vi "dataAcquisitionLoop.vi"(1 "total time":dbl format="%#_13g") -> (0 "Data Cluster":T1)   [LabVIEW 2013]
uses:
  <vilib>/Platform/TimedLoop/XDataNode/timing_clust.ctl
  <vilib>/Platform/TimedLoop/XDataNode/nitl_modes.ctl
  <vilib>/Platform/TimedLoop/XDataNode/wakeup.ctl
  <vilib>/DAQmx/read.llb/DAQmx Read (Analog 1D DBL NChan 1Samp).vi
  Global Variables.vi
  <vilib>/DAQmx/create/channels.llb/DAQmx Create Channel (AI-Voltage-Basic).vi
  <vilib>/DAQmx/configure/timing.llb/DAQmx Timing (Sample Clock).vi
  <vilib>/DAQmx/miscellaneous.llb/DAQmx Fill In Error Info.vi
  <vilib>/imath/engines/lvmath2/RunTimeEngine/NodeEndStatement/NIMS_NodeEndStatement_Output.vi
  <instcachedir>/0/NIMS_NodeEndStatement_Output_53EC0D466D134D7ABD903AC30B43404B.lvgen/NIMS_NodeEndStatement_Output_53EC0D466D134D7ABD903AC30B43404B_001.vi
  <vilib>/imath/engines/lvmath2/RunTimeEngine/ErrorHandling/NIMS_Finalize Error.vi
  <vilib>/Platform/TimedLoop/XDataNode/XDataNode.xnode
  <vilib>/Platform/TimedLoop/XDataNode/XDNodeRunTimeDep.lvlib
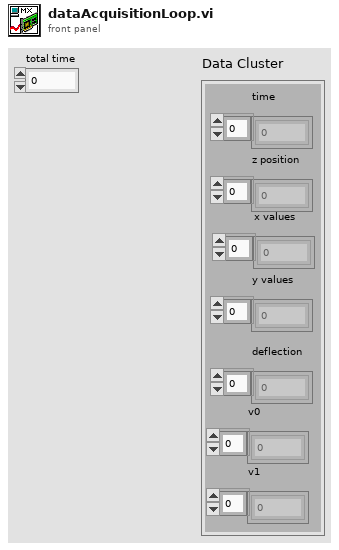
[diagram p1: front panel]
types:
  T1 = cluster{"time":dbl[], "z position":dbl[], "x values":dbl[], "y values":dbl[], "deflection":dbl[], "v0":dbl[], "v1":dbl[]}
  T2 = typedef "XDNodeRunTimeDep.lvlib/timing_clust.ctl" = cluster{"Expected End [f-1]":u64, "Actual End [f-1]":u64, "Finished Late? [f-1]":bool, "Expected End [i-1]":u64, "Actual End [i-1]":u64, "Finished Late? [i-1]":bool, "Expected Start [i]":u64, "Actual Start [i]":u64, "Expected Start [f]":u64, "Actual Start [f]":u64, "Source Name":string, "Structure Name":string, "Period":i64, "Deadline":i64, "Offset":i64, "Start":i64, "Priority":i32, "Timeout":i32, "Mode":T3, "Wakeup Reason":T4, "Error":errorcluster, "Source Type":string, "Secondary Source Type":string, "Global End Time":u64, "Global Start Time":u64, "Frame Duration":u64, "Iteration Duration":u64, "Assigned CPU":i32, "I/O Scan Engine Mode":u32}
  T3 = typedef "XDNodeRunTimeDep.lvlib/nitl_modes.ctl" = enum32{"No Change", "Process missed periods, maintain original phase", "Discard missed periods, maintain original phase", "Process missed periods, ignore original phase", "Discard missed periods, ignore original phase"}
  T4 = typedef "XDNodeRunTimeDep.lvlib/wakeup.ctl" = enum32{"Normal", "Aborted", "Asynchronous wakeup", "Timing source error", "Timed loop error", "Timeout"}
  T5 = cluster{dbl[], "flattned array":dbl[], dbl[], dbl[], "flattned array":dbl[], dbl[], dbl[]}
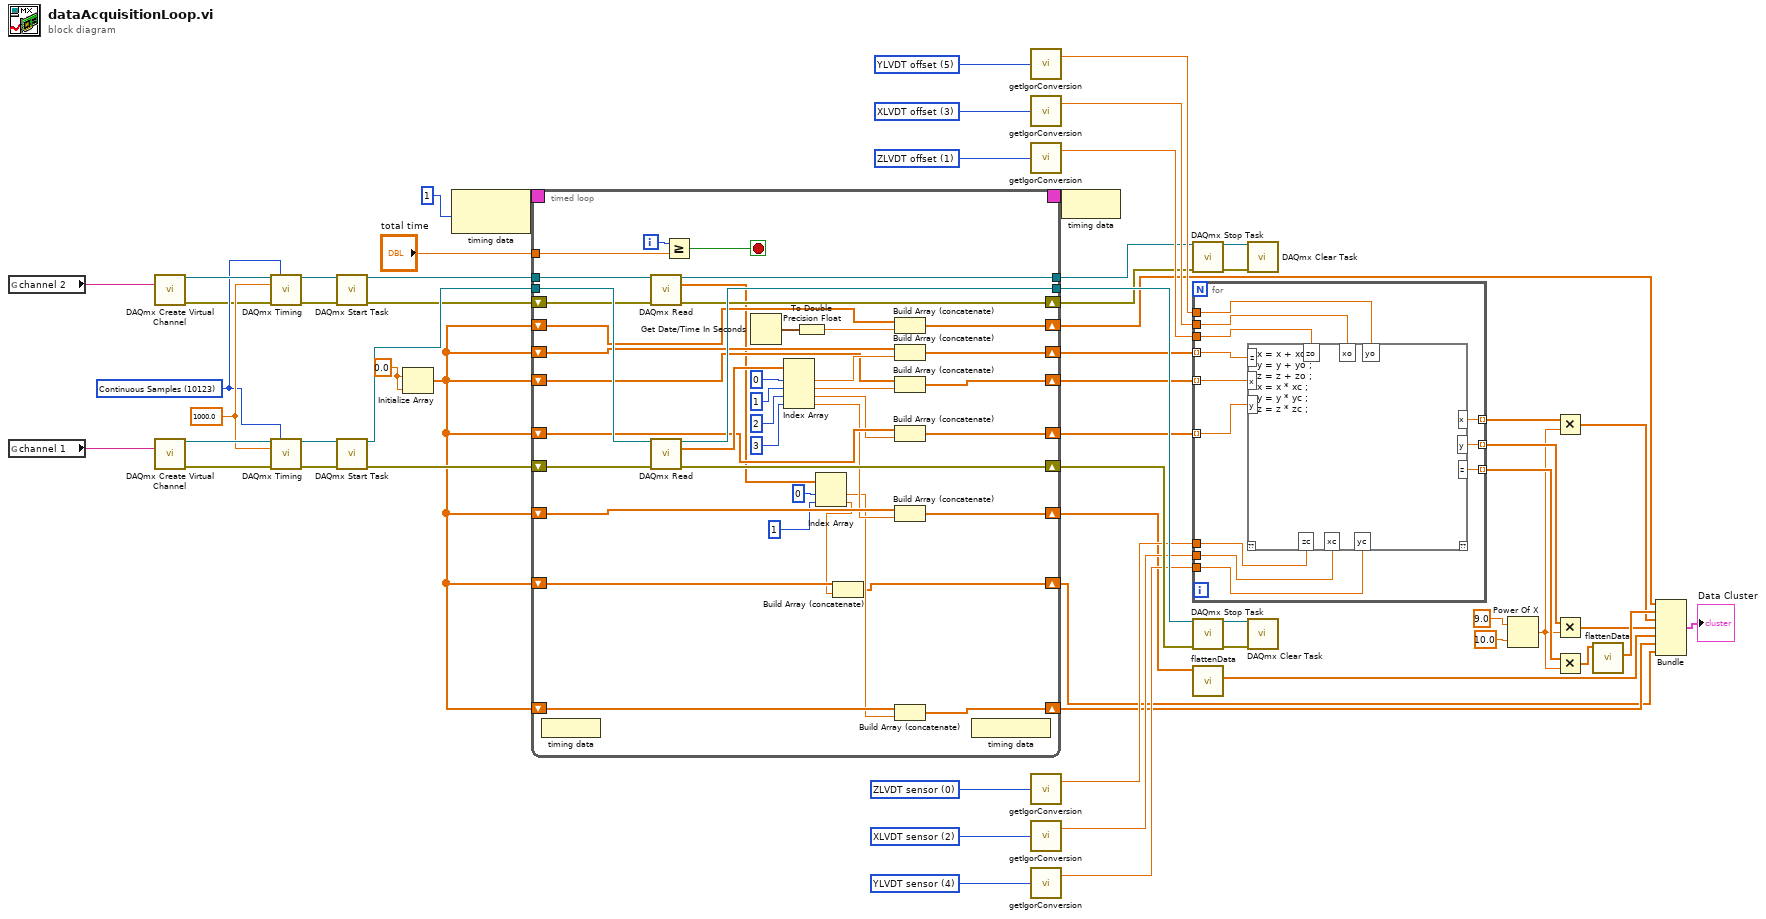
[diagram p0: block diagram]
diagram:
  w27 = 0.0
  w22 = 1000.0
  w34 = 1 items=["ZLVDT sensor", "ZLVDT offset", "XLVDT sensor", "XLVDT offset", "YLVDT sensor", "YLVDT offset", "DEFL"] ("index")
  w33 = 5 items=["ZLVDT sensor", "ZLVDT offset", "XLVDT sensor", "XLVDT offset", "YLVDT sensor", "YLVDT offset", "DEFL"] ("index")
  w32 = 3 items=["ZLVDT sensor", "ZLVDT offset", "XLVDT sensor", "XLVDT offset", "YLVDT sensor", "YLVDT offset", "DEFL"] ("index")
  w39 = 4 items=["ZLVDT sensor", "ZLVDT offset", "XLVDT sensor", "XLVDT offset", "YLVDT sensor", "YLVDT offset", "DEFL"] ("index")
  w38 = 2 items=["ZLVDT sensor", "ZLVDT offset", "XLVDT sensor", "XLVDT offset", "YLVDT sensor", "YLVDT offset", "DEFL"] ("index")
  w37 = 0 items=["ZLVDT sensor", "ZLVDT offset", "XLVDT sensor", "XLVDT offset", "YLVDT sensor", "YLVDT offset", "DEFL"] ("index")
  w19 = 10123 items=["Finite Samples"=10178, "Continuous Samples"=10123, "Hardware Timed Single Point"=12522] ("sample mode")
  n1 = global read "Global Variables.vi" "channel 2"() -> (w21:tag)
  n2 = global read "Global Variables.vi" "channel 1"() -> (w57:tag)
  n3 = call-poly <vilib>:"DAQmx Create Virtual Channel.vi"("physical channels"=w21) -> ("task out"=w20:refnum<k21>, "error out"=w18:errorcluster)  [unwired: 13 in]
  n4 = call-poly <vilib>:"DAQmx Create Virtual Channel.vi"("physical channels"=w57) -> ("task out"=w56:refnum<k21>, "error out"=w51:errorcluster)  [unwired: 13 in]
  n5 = call-poly <vilib>:"DAQmx Timing.vi"("task/channels in"=w20, "sample mode"=w19, "rate"=w22, "error in"=w18) -> ("task out"=w17:refnum<k21>, "error out"=w16:errorcluster)  [unwired: 10 in]
  n6 = call-poly <vilib>:"DAQmx Timing.vi"("task/channels in"=w56, "sample mode"=w19, "rate"=w22, "error in"=w51) -> ("task out"=w55:refnum<k21>, "error out"=w50:errorcluster)  [unwired: 10 in]
  n7 = call <vilib>:"DAQmx Start Task.vi"("task/channels in"=w17, "error in"=w16) -> ("task out"=w15:refnum<k21>, "error out"=w11:errorcluster)  [unwired: 12 in]
  n8 = call <vilib>:"DAQmx Start Task.vi"("task/channels in"=w55, "error in"=w50) -> ("task out"=w54:refnum<k21>, "error out"=w49:errorcluster)  [unwired: 12 in]
  n9 = Initialize Array(w27, w27) -> (w3:dbl[])
  n10 = node-c288(i64 1 ("Period")) -> (w61:T2)
  n11 = timed-loop {
    timing: w61 -> [_]
    timing-out: [_] -> w60
    tunnel: w54 -> [w102]
    tunnel: "total time" -> [w97]
    tunnel: [w101] -> w53
    shift-right: [w99] -> w48
    shift-left: w49 -> [w100]
    shift-right: [w89] -> w26
    shift-left: w3 -> [w90]
    shift-right: [w81] -> w23
    shift-left: w3 -> [w87]
    shift-right: [w79] -> w25
    shift-left: w3 -> [w85]
    shift-right: [w80] -> w24
    shift-left: w3 -> [w86]
    shift-right: [w77] -> w9
    shift-left: w3 -> [w78]
    tunnel: w15 -> [w74]
    tunnel: [w73] -> w13
    shift-right: [w71] -> w10
    shift-left: w11 -> [w72]
    shift-right: [w67] -> w4
    shift-left: w3 -> [w68]
    shift-right: [w62] -> w2
    shift-left: w3 -> [w64]
    i -> [w96]
    stop <- w98 stop-if-true
    n12 = node-c288() -> ()  [unwired: 1 in]
    n13 = call-poly <vilib>:"DAQmx Read.vi"("task/channels in"=w74, "error in"=w72) -> ("task out"=w73:refnum<k21>, "data"=w70:dbl[], "error out"=w71:errorcluster)  [unwired: 11 in]
    n14 = call-poly <vilib>:"DAQmx Read.vi"("task/channels in"=w102, "error in"=w100) -> ("task out"=w101:refnum<k21>, "data"=w95:dbl[], "error out"=w99:errorcluster)  [unwired: 11 in]
    n15 = Greater Or Equal?(x=w96, y=w97) -> (x >= y?=w98:bool)
    n16 = Get Date/Time In Seconds() -> (seconds since 1Jan1904=w76:timestamp)
    n17 = Index Array(array=w95, index #1=0, index #2=1, index #3=2, index #4=3) -> (element #1=w88:dbl, element #2=w84:dbl, element #3=w83:dbl, element #4=w82:dbl)
    n18 = To Double Precision Float(number=w76) -> (double precision float=w75:dbl)
    n19 = Index Array(array=w70, index #1=0, index #2=1) -> (element #1=w66:dbl, element #2=w63:dbl)
    n20 = Build Array (concatenate)(w64, w63) -> (w62:dbl[])
    n21 = Build Array (concatenate)(w78, w75) -> (w77:dbl[])
    n22 = Build Array (concatenate)(w90, w88) -> (w89:dbl[])
    n23 = Build Array (concatenate)(w85, w84) -> (w79:dbl[])
    n24 = Build Array (concatenate)(w86, w83) -> (w80:dbl[])
    n25 = Build Array (concatenate)(w87, w82) -> (w81:dbl[])
    n26 = Build Array (concatenate)(w68, w66) -> (w67:dbl[])
    n27 = node-c288() -> ()  [unwired: 1 out]
  }
  n28 = call "getIgorConversion.vi"("index"=w33) -> ("Result"=w31:dbl)  [unwired: 1 out]
  n29 = call "getIgorConversion.vi"("index"=w32) -> ("Result"=w30:dbl)  [unwired: 1 out]
  n30 = call "getIgorConversion.vi"("index"=w34) -> ("Result"=w29:dbl)  [unwired: 1 out]
  n31 = call "getIgorConversion.vi"("index"=w37) -> ("Result"=w28:dbl)  [unwired: 1 out]
  n32 = call "getIgorConversion.vi"("index"=w38) -> ("Result"=w36:dbl)  [unwired: 1 out]
  n33 = call "getIgorConversion.vi"("index"=w39) -> ("Result"=w35:dbl)  [unwired: 1 out]
  n34 = node-c288(w60) -> ()
  n35 = call <vilib>:"DAQmx Stop Task.vi"("task/channels in"=w13, "error in"=w10) -> ("task out"=w12:refnum<k21>, "error out"=w14:errorcluster)  [unwired: 12 in]
  n36 = for {
    tunnel: w26 -> [w105] mode=indexing
    tunnel: w25 -> [w106] mode=indexing
    tunnel: w24 -> [w107] mode=indexing
    tunnel: [w116] -> w42 mode=indexing
    tunnel: [w115] -> w43 mode=indexing
    tunnel: [w114] -> w44 mode=indexing
    tunnel: w28 -> [w113]
    tunnel: w36 -> [w112]
    tunnel: w35 -> [w111]
    tunnel: w31 -> [w110]
    tunnel: w30 -> [w109]
    tunnel: w29 -> [w108]
    n37 = mathscript code="x = x + xo ;\ny = y + yo ;\nz = z + zo ;\nx = x * xc ;\ny = y * yc ;\nz = z * zc ;"("x"=w106, "y"=w107, "z"=w105, "zo"=w108, "yo"=w110, "xo"=w109, "zc"=w113, "xc"=w112, "yc"=w111) -> ("x"=w114:dbl, "y"=w115:dbl, "z"=w116:dbl)  [unwired: 1 in, 1 out]
  }
  n38 = call <vilib>:"DAQmx Stop Task.vi"("task/channels in"=w53, "error in"=w48) -> ("task out"=w52:refnum<k21>, "error out"=w47:errorcluster)  [unwired: 12 in]
  n39 = call "flattenData.vi"("input array"=w23) -> ("flattned array"=w5:dbl[])  [unwired: 9 in, 1 out]
  n40 = call <vilib>:"DAQmx Clear Task.vi"("task in"=w12, "error in"=w14) -> ()  [unwired: 13 in, 1 out]
  n41 = call <vilib>:"DAQmx Clear Task.vi"("task in"=w52, "error in"=w47) -> ()  [unwired: 13 in, 1 out]
  n42 = Power Of X(1:10.0 ("x"), 2:9.0 ("y")) -> (0:w41:dbl)
  n43 = Multiply(x=w44, y=w41) -> (x*y=w7:dbl[])
  n44 = Multiply(x=w43, y=w41) -> (x*y=w6:dbl[])
  n45 = Multiply(x=w42, y=w41) -> (x*y=w40:dbl[])
  n46 = call "flattenData.vi"("input array"=w40) -> ("flattned array"=w8:dbl[])  [unwired: 9 in, 1 out]
  n47 = Bundle(w9, "flattned array"=w8, w7, w6, "flattned array"=w5, w4, w2) -> (→"Data Cluster":T5)  [unwired: 1 in]
